vi "Untitled 5.vi"(8 "error in":errorcluster, 11 "StellarNetSpecAcquisition in":refnum<class "StellarNetSpecAcquisition.lvclass">) -> (0 "error out":errorcluster, 3 "StellarNetSpecAcquisition out":refnum<class "StellarNetSpecAcquisition.lvclass">)   [LabVIEW 2013, in "StellarNetSpecAcquisition.lvclass"]
uses:
  StellarNetSpecAcquisition.lvclass
  StellarNetSpecAcquisition.lvclass/StellarNetSpecAcquisition.ctl
  StellarNetSpectrometerClass/StellarNetSpectrometer.lvclass
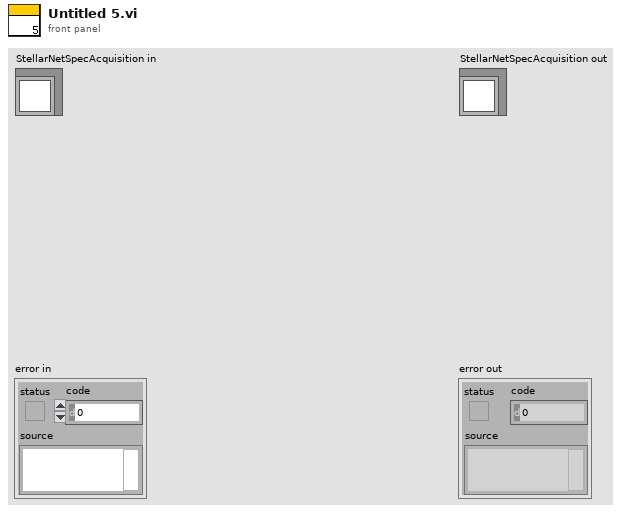
[diagram p1: front panel]
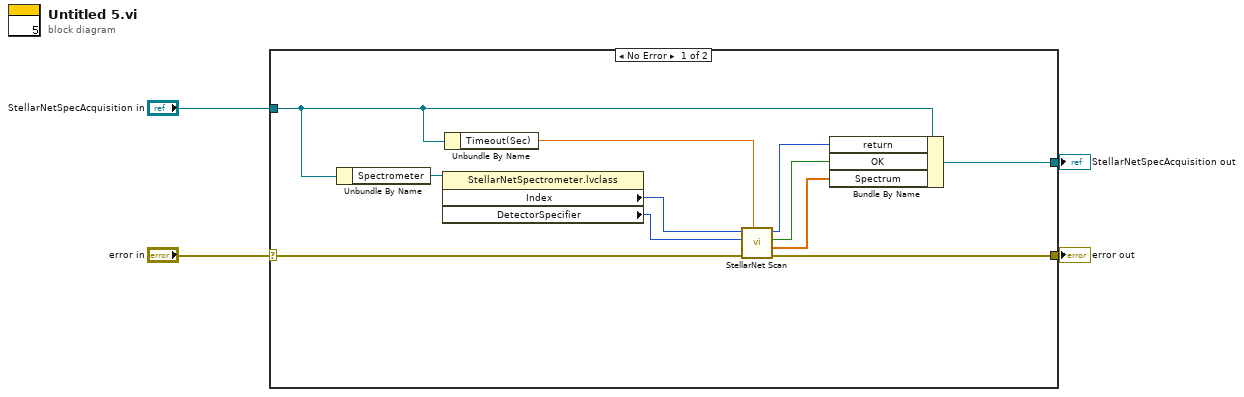
[diagram p0: block diagram]
diagram:
  n1 = case shown="No Error" "error in" {
    selector: "error in" -> [w12 w17]
    tunnel: [w11 w17] -> w3
    tunnel: [w5 w16] -> w1
    tunnel: "StellarNetSpecAcquisition in" -> [w6 w16]
    frame No Error {
      n2 = Unbundle By Name(w6) -> ("Spectrometer"=w15:refnum<class "StellarNetSpectrometer.lvclass">)
      n3 = property class="StellarNetSpectrometer.lvclass"(reference=w15) -> ("Index"=w14:u32, "DetectorSpecifier"=w13:u16)  [unwired: 1 in, 2 out]
      n4 = Unbundle By Name(w6) -> ("Timeout(Sec)"=w10:dbl)
      n5 = call "StellarNet Scan.vi"("Timeout(Sec)"=w10, "error in"=w12, "DetectorSpecifier"=w13, "Index"=w14) -> ("error out"=w11:errorcluster, "Spectrum"=w7:sgl[], "OK"=w8:bool, "return"=w9:i32)  [unwired: 4 in]
      n6 = Bundle By Name(cluster=w6, "return"=w9, "OK"=w8, "Spectrum"=w7) -> (w5:refnum<class "StellarNetSpecAcquisition.lvclass">)
    }
    frame Error {
    }
  }
  "error out" <- w3
  "StellarNetSpecAcquisition out" <- w1
